vi "Image Data to RGB.vi"(0 "image data":T1, 5 "error in (no error)":errorcluster) -> (14 "Image_3d_RGB":u8[][][](array[numeric]), 19 "error out":errorcluster)   [LabVIEW 2015]
uses:
  <vilib>/picture/picture.llb/imagedata.ctl
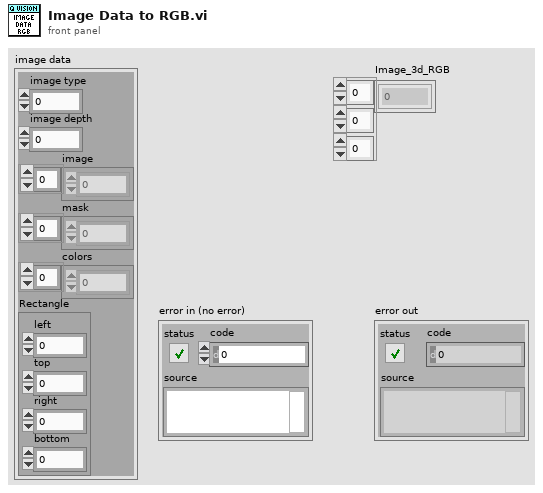
[diagram p1: front panel]
types:
  T1 = typedef "imagedata.ctl" = cluster{"image type":i32, "image depth":i32, "image":u8[], "mask":u8[], "colors":u32[], "Rectangle":cluster{"left":i16, "top":i16, "right":i16, "bottom":i16}}
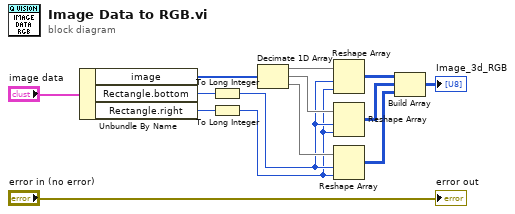
[diagram p0: block diagram]
diagram:
  n1 = Unbundle By Name("image data") -> ("image"=w13:u8[], "Rectangle.bottom"=w9:i16, "Rectangle.right"=w8:i16)
  n2 = To Long Integer(number=w9) -> (32bit integer=w7:i32)
  n3 = To Long Integer(number=w8) -> (32bit integer=w6:i32)
  n4 = Decimate 1D Array(w13) -> (w12:u8[], w11:u8[], w10:u8[])
  n5 = Reshape Array(w12, w7, w6) -> (w5:u8[][])
  n6 = Reshape Array(w11, w7, w6) -> (w4:u8[][])
  n7 = Reshape Array(w10, w7, w6) -> (w3:u8[][])
  n8 = Build Array(w5, w4, w3) -> (→"Image_3d_RGB":u8[][][])
  "error out" <- "error in (no error)"
